vi "MU Calibration Is Analog Analyze Result Adjustable.vi"(7 "adjustmentMessageLogLevel":u32, 8 "error in (no error)":errorcluster, 9 "adjustmentMessageBufferSize":u64=1024, 10 "analyzeResult":T2, 11 "CalibrationHandle":T1) -> (0 "error out (no error)":errorcluster, 2 "adjustMessage":string, 3 "Result":bool)   [LabVIEW 2017, in "MU_3SL_interface.lvlib"]
uses:
  MU_3SL_interface.lvlib
  handles/CalibrationAnalyzeResultHandle.ctl
  handles/CalibrationHandle.ctl
  lib/MU_3SL_interface.dll
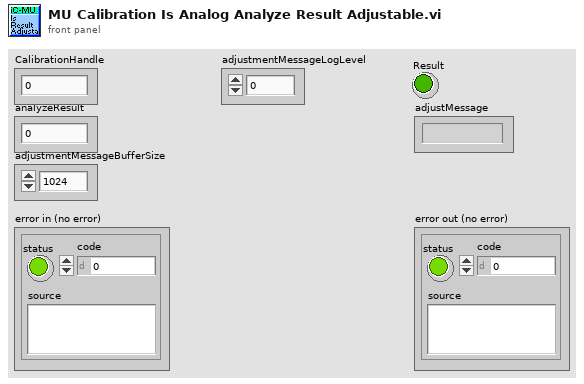
[diagram p1: front panel]
types:
  T1 = typedef "MU_3SL_interface.lvlib/CalibrationHandle.ctl" = u64
  T2 = typedef "MU_3SL_interface.lvlib/CalibrationAnalyzeResultHandle.ctl" = u64
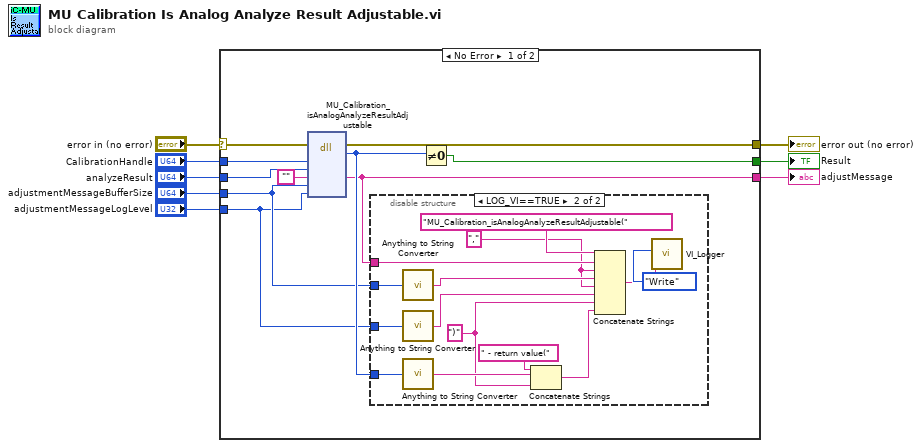
[diagram p0: block diagram]
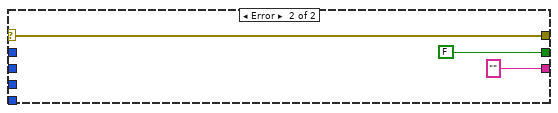
[diagram p3: hidden frame]
diagram:
  n1 = case shown="No Error" "error in (no error)" {
    selector: "error in (no error)" -> [w18 w35]
    tunnel: [w16 w35] -> w8
    tunnel: "analyzeResult" -> [w17 _]
    tunnel: [w15 FALSE] -> w5
    tunnel: [w12 "" ("adjustMessage")] -> w4
    tunnel: "CalibrationHandle" -> [w14 _]
    tunnel: "adjustmentMessageBufferSize" -> [w11 _]
    tunnel: "adjustmentMessageLogLevel" -> [w10 _]
    frame No Error {
      n2 = dll-call lib="C:/Users/bes/AppData/Roaming/work/mu_9so/icsubmodules/soft_mu_3sl_master/lv_interface/lib/MU_3SL_interface**.*" fn="MU_Calibration_isAnalogAnalyzeResultAdjustable"(error in=w18, "calibrationHandle"=w14, "analyzeResultHandle"=w17, "adjustMessage"="", "adjustmentMessageBufferSize"=w11, "adjustmentMessageLogLevel"=w10) -> (error out=w16:errorcluster, "return type"=w13:u8, "adjustMessage"=w12:string)  [unwired: 6 in, 1 out]
      n3 = disable-structure shown="LOG_VI==TRUE" {
        disable-tunnel: w13 -> [_ w28]
        disable-tunnel: w12 -> [_ w26]
        disable-tunnel: w11 -> [_ w25]
        disable-tunnel: w10 -> [_ w24]
        frame condition #0 {
        }
        frame condition #1 (active) {
          w22 = "," ("string")
          w20 = ")" ("string")
          n4 = call "Anything to String Converter.vi"("anything"=w25) -> ("String"=w23:string)
          n5 = call "Anything to String Converter.vi"("anything"=w24) -> ("String"=w21:string)
          n6 = call "Anything to String Converter.vi"("anything"=w28) -> ("String"=w27:string)
          n7 = Concatenate Strings(" - return value(" ("string"), w27, w20) -> (w19:string)
          n8 = Concatenate Strings("MU_Calibration_isAnalogAnalyzeResultAdjustable(" ("Info in"), w26, w22, w23, w22, w21, w20, w19) -> (w30:string)
          n9 = call "VI_Logger.vi"("Action (Read)"=enum16{"Write", "Read"}."Write", "Info in"=w30) -> ()  [unwired: 8 in, 2 out]
        }
      }
      n10 = Not Equal To 0?(x=w13) -> (x != 0?=w15:bool)
    }
    frame Error {
    }
  }
  "error out (no error)" <- w8
  "Result" <- w5
  "adjustMessage" <- w4
